vi "SigCheck.vi"(11 "Path":path) -> (3 "standard output":string)   [LabVIEW 2014, in "application.lvclass"]
uses:
  application.lvclass
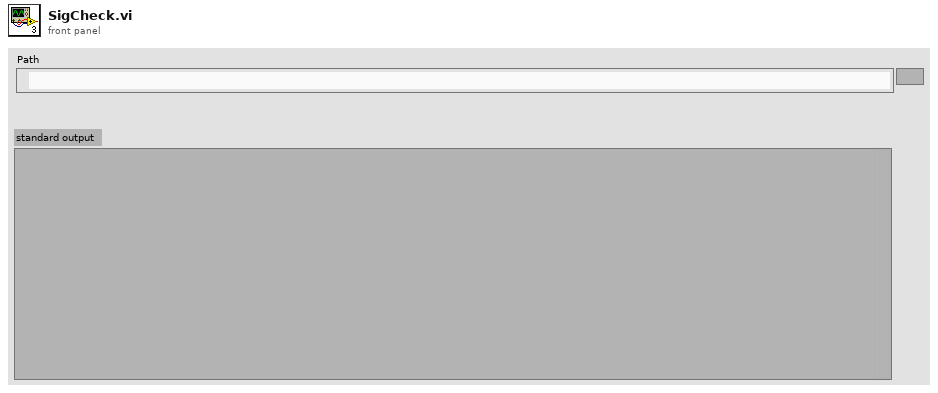
[diagram p1: front panel]
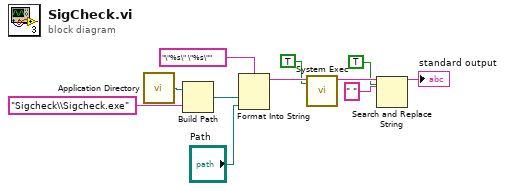
[diagram p0: block diagram]
diagram:
  n1 = call <vilib>:"Application Directory.vi"() -> ("Application Directory"=w11:path)
  n2 = Build Path(base path=w11, name or relative path="Sigcheck\\Sigcheck.exe") -> (appended path=w9:path)
  n3 = Format Into String(format string="\"%s\" \"%s\"", w9, "Path") -> (resulting string=w7:string)  [unwired: 2 in, 1 out]
  n4 = call <vilib>:"System Exec.vi"("wait until completion? (T)"=TRUE, "command line"=w7) -> ("standard output"=w4:string)  [unwired: 6 in, 3 out]
  n5 = Search and Replace String(replace all?=TRUE ("replace all? (F)"), input string=w4, search string=" ") -> (result string=→"standard output":string)  [unwired: 5 in, 3 out]
